vi "MasterAquisitionFile_IOS_postCleanUp.vi"() -> ()   [LabVIEW 2017]
uses:
  <vilib>/userdefined/High Color/IMAQdx.ctl
  <vilib>/vision/driver/IMAQdx.llb/IMAQdx Acquisition Mode.ctl
  <vilib>/vision/driver/IMAQdx.llb/IMAQdx Camera Control Mode.ctl
  <vilib>/vision/driver/IMAQdx.llb/IMAQdx Buffer Number Mode.ctl
  <vilib>/DAQmx/write.llb/DAQmx Write (Digital Bool 1Line 1Point).vi
  <vilib>/DAQmx/read.llb/DAQmx Read (Analog 1D Wfm NChan NSamp).vi
  <vilib>/DAQmx/write.llb/DAQmx Write (Digital 1D Bool NChan 1Samp 1Line).vi
  <vilib>/DAQmx/create/channels.llb/DAQmx Create Channel (DO-Digital Output).vi
  <vilib>/DAQmx/create/channels.llb/DAQmx Create Channel (CO-Pulse Generation-Frequency).vi
  <vilib>/DAQmx/configure/timing.llb/DAQmx Timing (Implicit).vi
  <vilib>/DAQmx/create/channels.llb/DAQmx Create Channel (AI-Voltage-Basic).vi
  <vilib>/DAQmx/configure/timing.llb/DAQmx Timing (Sample Clock).vi
  <vilib>/DAQmx/configure/trigger.llb/DAQmx Start Trigger (Digital Edge).vi
  <vilib>/DAQmx/miscellaneous.llb/DAQmx Fill In Error Info.vi
  <vilib>/vision/driver/NI_Vision_Acquisition_Software.lvlib
  <resource>/objmgr/imaqdx.rc
panel:
  in  "Exposure Time (microsec)":string="10000"
  out "Dropped Frame Table":string[][](table)=[["1236", "1"], ["15481", "1"], ["43559", "1"]]
  out "Solenoids":bool[](array[boolean])
  out "Whisker Camera":bool
  out "Analog Data":bool
  out "Analog acquisition length":i32=61960
  in  "Channel Labels":string[](array[string])=["Neural_LH", "Force_Sensor", "Solenoid_LeftPad", "Solenoid_RightPad", "Solenoid_Auditory", "Respiration", "EMG", "Neural_RH"]
  in  "physical channels":tag="Dev1/ai0:7"
  in  "Whisker Cam ID":T1="cam0"
  in  "WebCam ID":T1="cam3"
  in  "Analog Acquisition":cluster{"Analog Sampling Rate":u16}={"Analog Sampling Rate"=20000} {"Analog Sampling Rate" format="%0.0f"}
  in  "Camera Acquisition Setup":T2={"CBVCam Rate"=30, "WhiskerCam Rate"=150, "WebCam Rate"=15}
  out "Notes Size":i32=7
  out "Notes Reversed":string[](array[string])=["Experimenter", "Animal ID", "Imaged Hemisphere", "Solenoid Pressure", "Isoflurane time", "Session ID", "Amplifier Gain"]
  out "Notes Array":string[](array[string])=["Amplifier Gain", "Session ID", "Isoflurane time", "Solenoid Pressure", "Imaged Hemisphere", "Animal ID", "Experimenter"]
  in  "Session Notes:":T3={"Experimenter"="Kevin", "Animal ID"="T70", "Imaged Hemisphere"="Both", "Solenoid Pressure"="10", "Isoflurane time"="1350", "Session ID"="ImagingSessionOne", "Amplifier Gain"="10000"}
  in  "WhiskCam Trig Source":tag="Dev1/ctr1"
  in  "CBV Cam Trig Source":tag="Dev1/ctr0"
  in  "Left Pad":tag="Dev1/port0/line1"
  in  "Right Pad":tag="Dev1/port0/line0"
  in  "Auditory":tag="Dev1/port0/line3"
  in  "Tail":tag="Dev1/port0/line2"
  in  "Stim Offset (s)":dbl=15.0
  in  "Stim Duration (s)":dbl=0.1 step=0.1
  in  "Inter-Stim Interval (s)":dbl=30.0
  in  "Left Pad":dbl=1.0
  in  "Right Pad":dbl=1.0
  in  "Auditory":dbl=1.0
  in  "Tail":dbl
  in  "Target Path":path=path "C:/Users/klt8/Documents" caption="Final saved file location"
  out "Dropped":u32(slide) caption="Dropped Whisker\nCamera Frames" scale=0.0..50.0
  out "Current file name":string="190407_21_19_47"
  out "Actual WebCam Frame Rate":dbl(knob) scale=0.0..30.0
  out "WebCam":T4(plugin-control)
  out "CBV Camera":bool
  out "Trial Time Elapsed (Min)":cluster{dbl, dbl}(slide)={5.0, 0.051677} scale=0.0..5.0
  in  "Recording Time (min)":dbl(knob)=5.0 min=0.5 max=10.0 step=0.5 scale=0.0..5.0 scale format="%#_2g"
  in  "Temp Path":path=path "C:/Users/klt8/Documents/LabView Test Files" caption="Temporary path for\nstreamed data"
  out "Last CBV\nBuffer":i32=92
  in  "Stop":bool
  out "Actual CBVCam\nFrame Rate":dbl(knob)=30.0 scale=0.0..100.0
  out "Last Whisk\nBuffer":u32=463
  out "Actual WhiskCam\nFrame Rate":dbl(knob)=150.0 scale=0.0..300.0
  # "# Dropped"
  # "Dropped\nIndex"
  # "File Settings:"
  # "Right Pad"
  # "Left Pad"
  # "Tail"
  # "Auditory"
  # "Stimulation Settings:"
  # "Stim. Ratios:"
  # "Output Channels:"
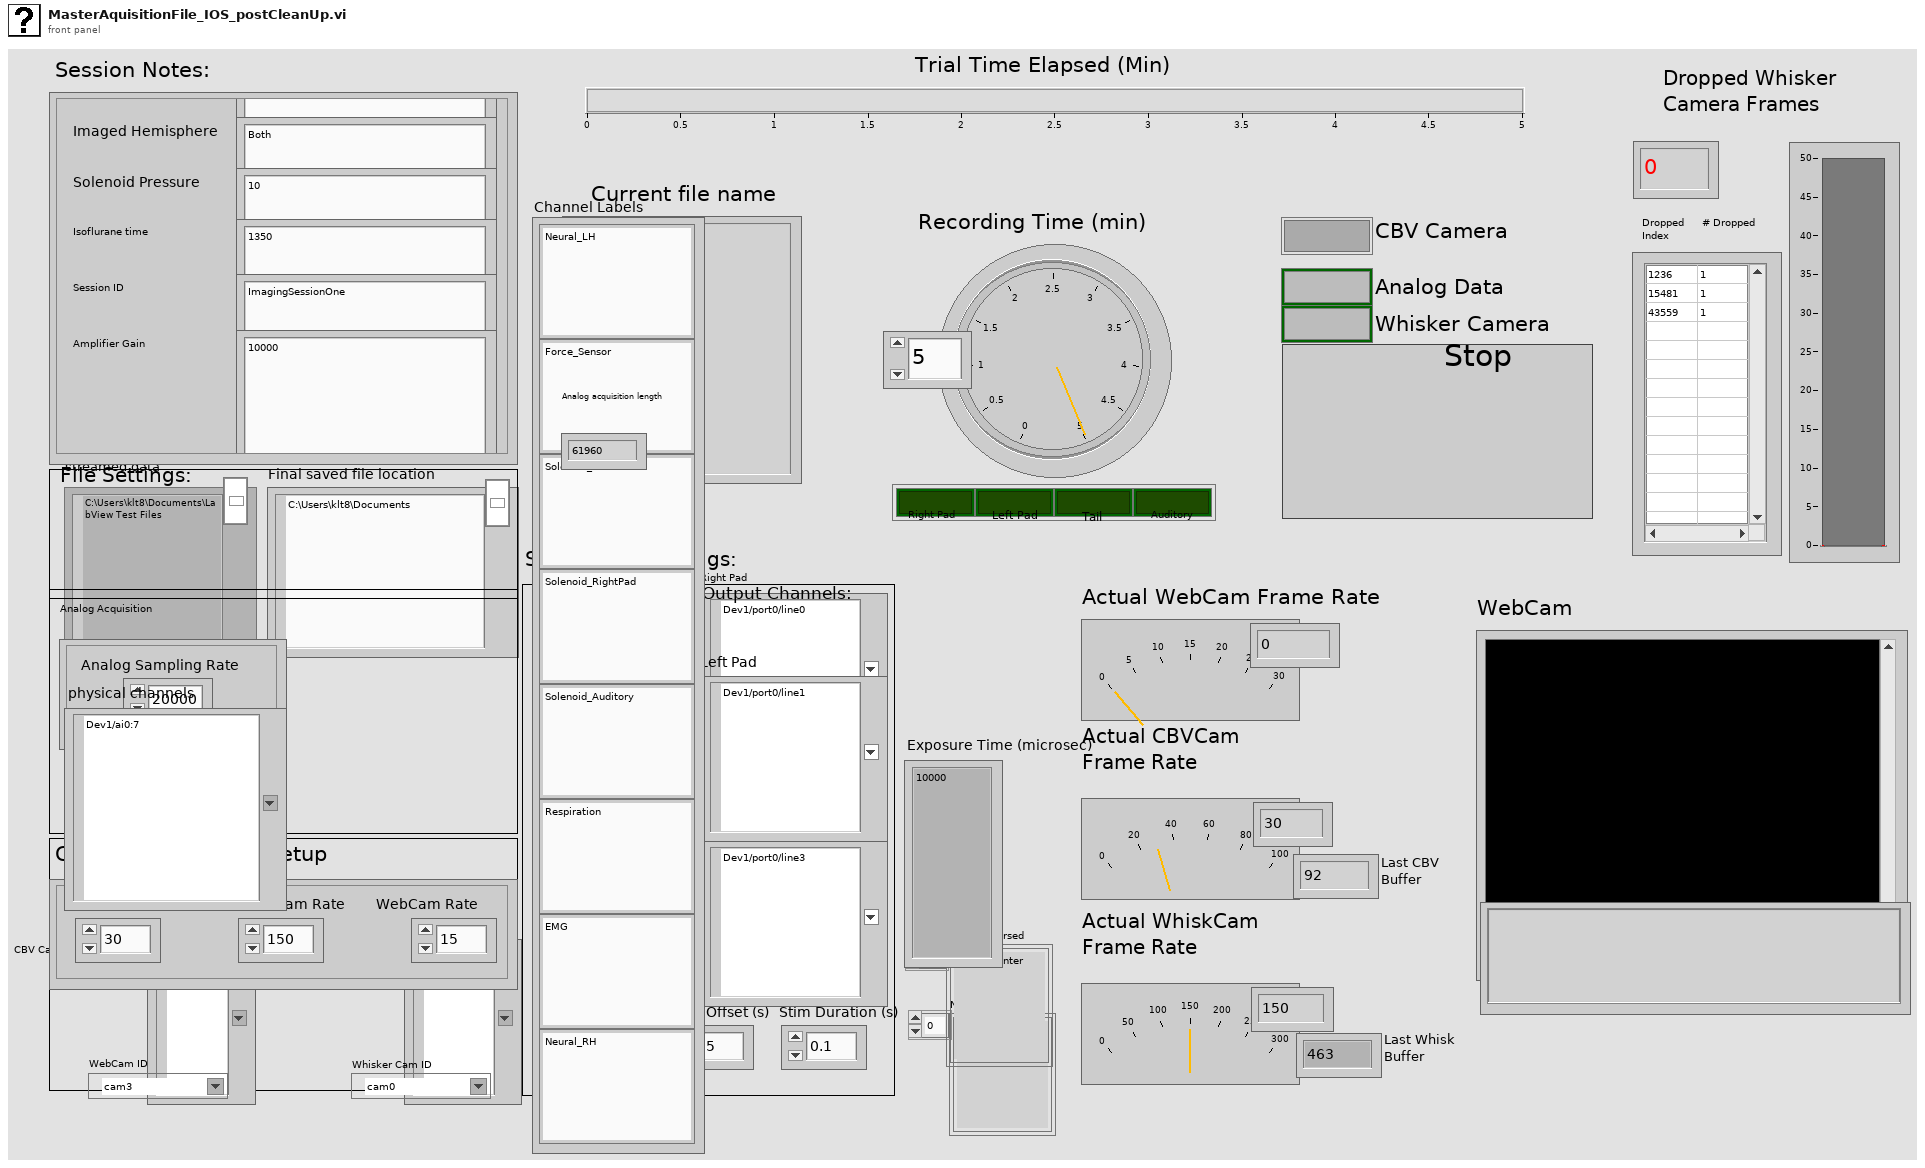
[diagram p1: front panel]
types:
  T1 = typedef "IMAQdx.ctl" = refnum<k21>
  T2 = cluster{"CBVCam Rate":u16, "WhiskerCam Rate":u16, "WebCam Rate":u16}
  T3 = cluster{"Experimenter":string, "Animal ID":string, "Imaged Hemisphere":string, "Solenoid Pressure":string, "Isoflurane time":string, "Session ID":string, "Amplifier Gain":string}
  T4 = typedef "IMAQ Image.ctl" = refnum<image>
  T5 = enum16{"open", "open or create", "create or replace", "create", "open (read-only)"}
  T6 = typedef "Image Type" = u32
  T7 = typedef "NI_Vision_Acquisition_Software.lvlib/IMAQdx Camera Control Mode.ctl" = enum32{"Controller", "Listener"}
  T8 = enum16{"open", "replace", "create", "open or create", "replace or create", "replace or create with confirmation"}
  T9 = typedef "NI_Vision_Acquisition_Software.lvlib/IMAQdx Acquisition Mode.ctl" = enum32{"One Shot", "Continuous"}
  T10 = typedef "IMAQ AVI2 Refnum.ctl" = refnum<k20>
  T11 = enum16{"big-endian, network order", "native, host order", "little-endian"}
  T12 = typedef "NI_Vision_Acquisition_Software.lvlib/IMAQdx Buffer Number Mode.ctl" = enum32{"Next", "Last", "Buffer Number", "Every", "Last New"}
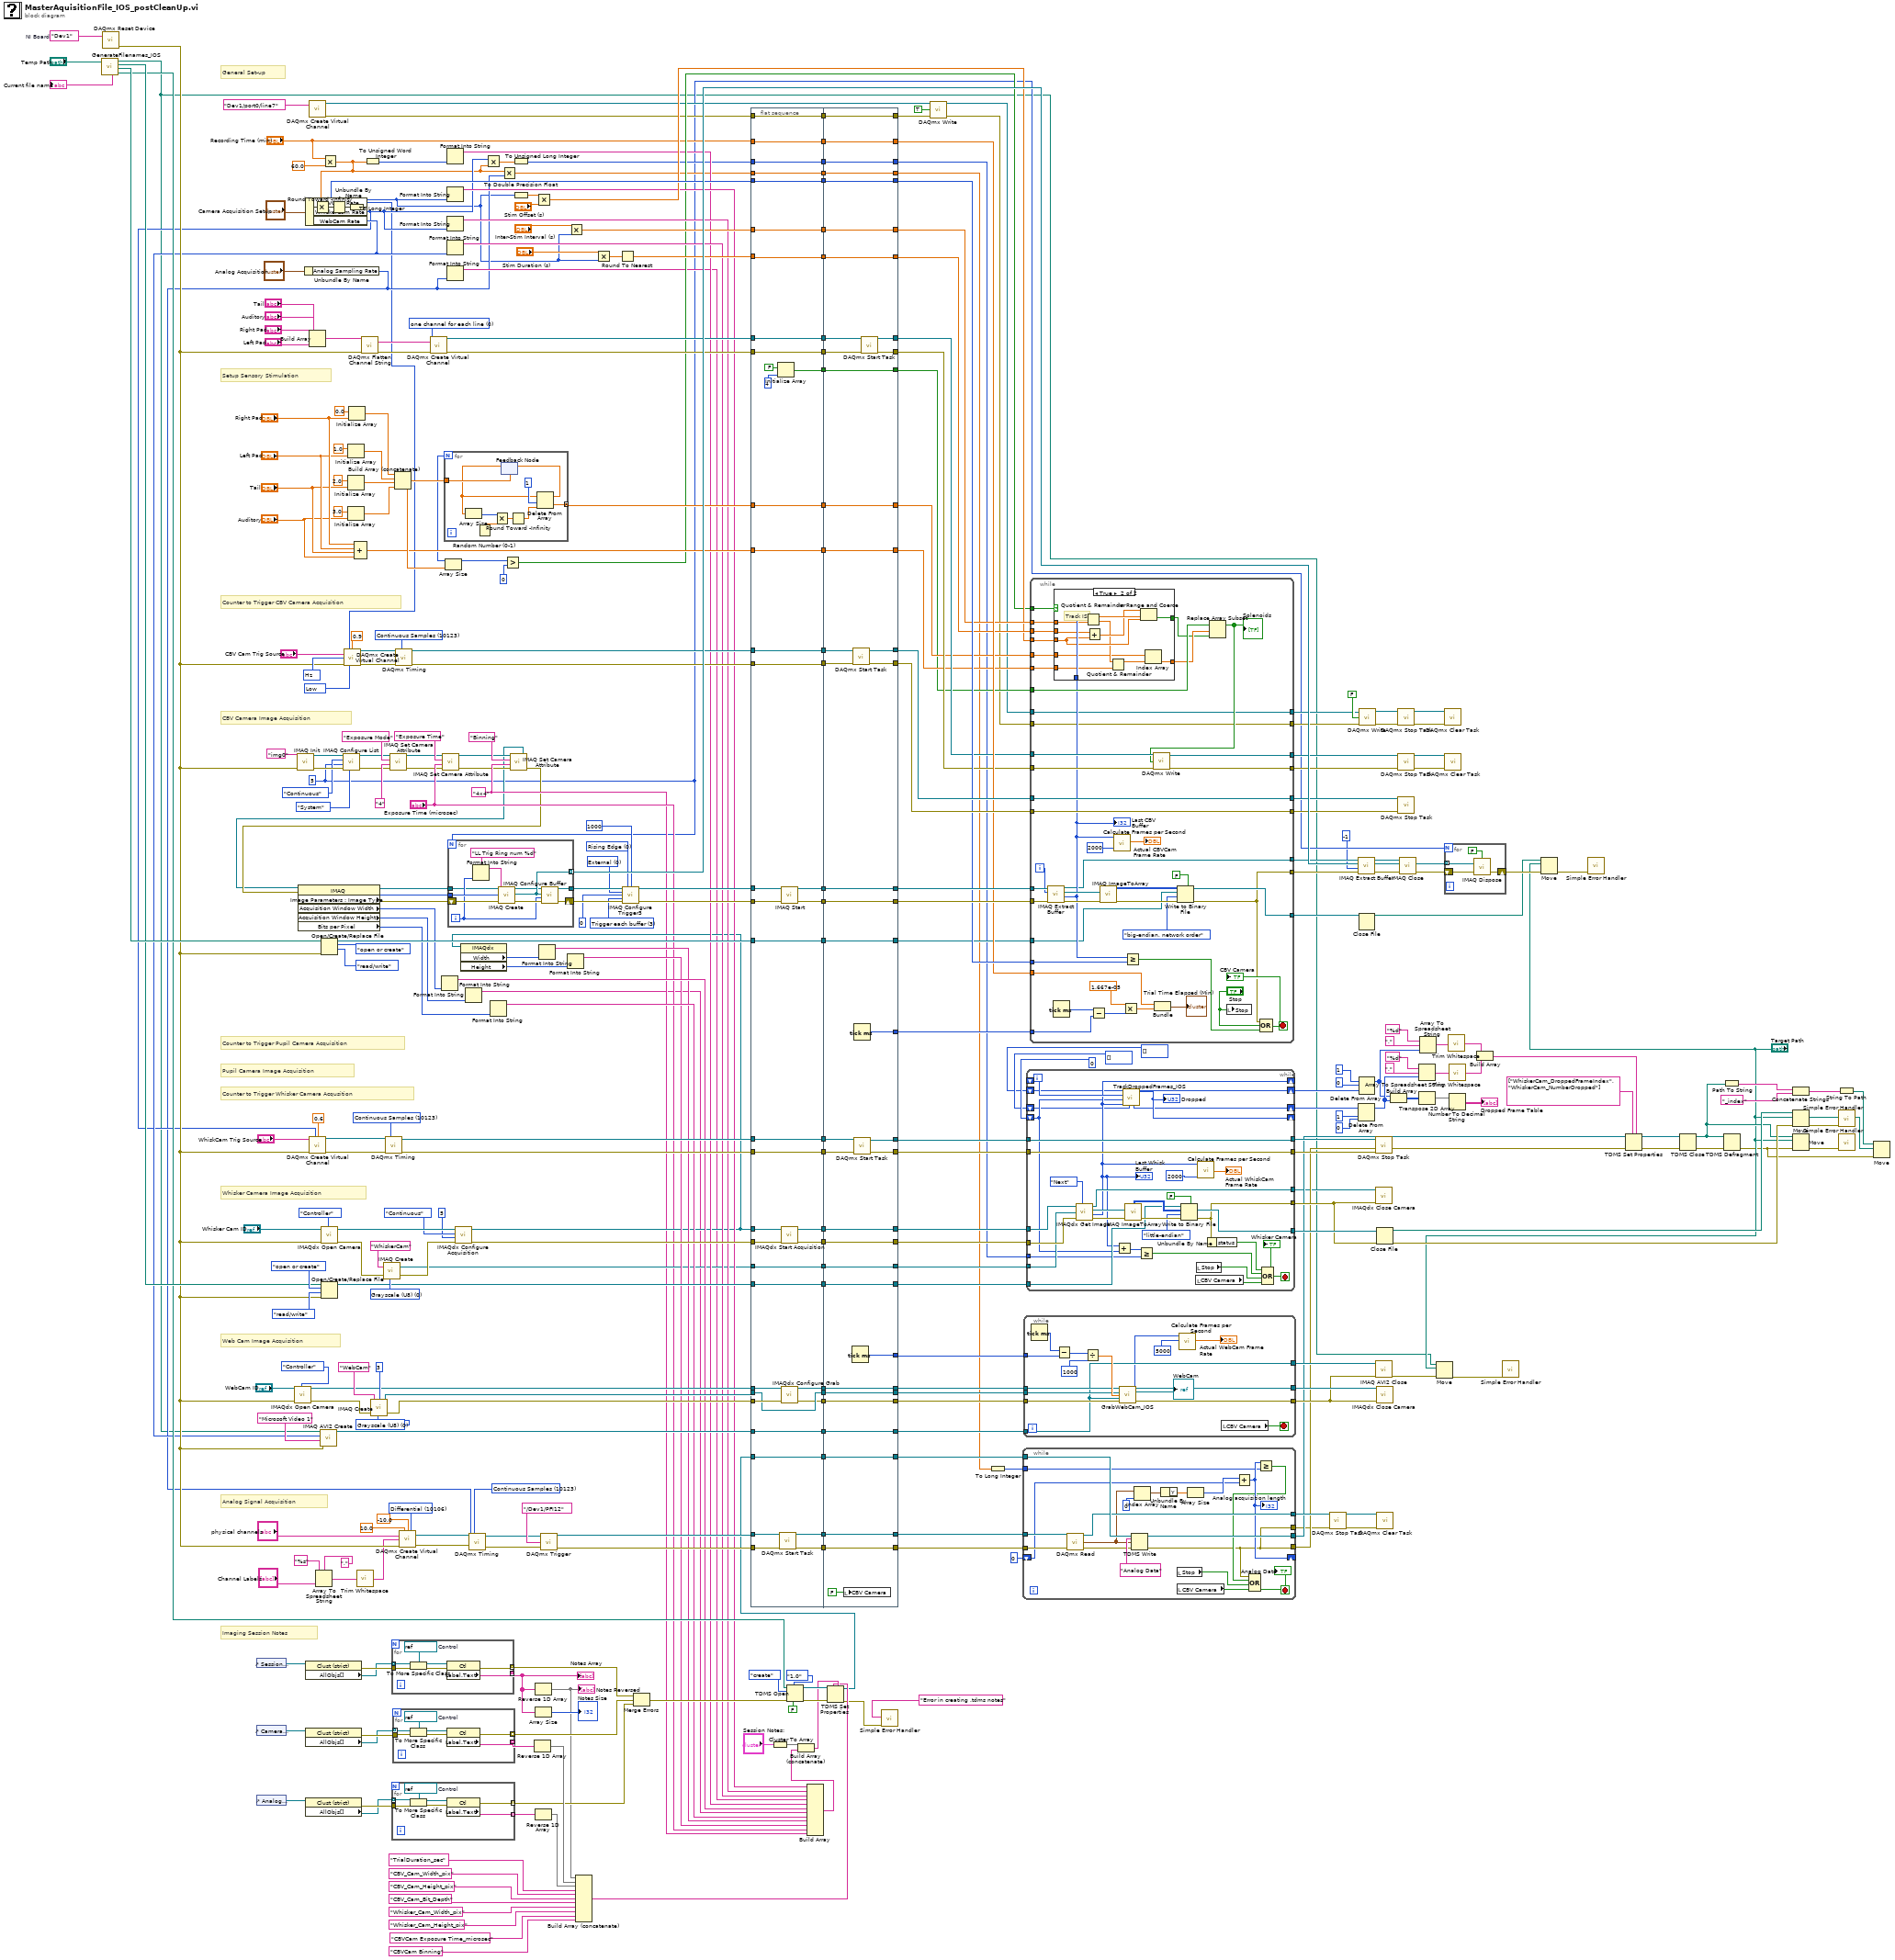
[diagram p0: block diagram]
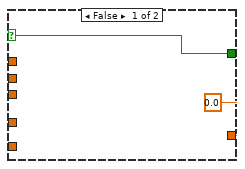
[diagram p2: hidden frame]
diagram:
  w34 = "4x4" ("Attribute Value")
  w195 = 0 items=["one channel for each line", "one channel for all lines"] ("line grouping")
  w252 = 10123 items=["Finite Samples"=10178, "Continuous Samples"=10123, "Hardware Timed Single Point"=12522] ("sample mode")
  w255 = 10106 items=["default"=-1, "RSE"=10083, "NRSE"=10078, "Differential"=10106, "Pseudodifferential"=12529] ("input terminal configuration")
  w309 = T6 0 items=["Grayscale (U8)", "Grayscale (I16)", "Grayscale (SGL)", "Complex (CSG)", "RGB (U32)", "HSL (U32)", "RGB (U64)", "Grayscale (U16)"] ("Image Type")
  w329 = u32 0 items=["Rising Edge", "Falling Edge"] ("Trigger Polarity")
  w332 = u32 0 items=["External"=0, "RTSI"=1, "ISO In"=2, "Scaled Encoder"=5] ("Trigger Type")
  w323 = tag "Dev1"  # NI Board
  w324 = 10123 items=["Finite Samples"=10178, "Continuous Samples"=10123, "Hardware Timed Single Point"=12522] ("sample mode")
  w327 = 10373 items=["Hz"=10373] ("units")
  w328 = 10214 items=["High"=10192, "Low"=10214] ("idle state")
  w5 = u32 5 ("Number of Buffers")
  w330 = u32 3 items=["Disabled", "Trigger start of acquisition", "Trigger start of each buffer list", "Trigger each buffer", "Trigger each line (linescan)", "Trigger end of acquisition"] ("Action")
  w344 = 10123 items=["Finite Samples"=10178, "Continuous Samples"=10123, "Hardware Timed Single Point"=12522] ("sample mode")
  w351 = T6 0 items=["Grayscale (U8)", "Grayscale (I16)", "Grayscale (SGL)", "Complex (CSG)", "RGB (U32)", "HSL (U32)", "RGB (U64)", "Grayscale (U16)"] ("Image Type")
  # "General Set-up"
  # "Pupil Camera Image Acquisition"
  # "Counter to Trigger Pupil Camera Acquisition"
  # "Whisker Camera Image Acquisition"
  # "Imaging Session Notes"
  # "Setup Sensory Stimulation"
  # "CBV Camera Image Acquisition"
  # "Counter to Trigger CBV Camera Acquisition"
  # "Counter to Trigger Whisker Camera Acqusition"
  # "Web Cam Image Acquisition"
  # "Analog Signal Acquisition"
  n1 = call "GenerateFilenames_IOS.vi"("path"="Temp Path") -> ("TDMS Path"=w144:path, "Dalsa Path"=w316:path, "Basler Path"=w312:path, "WebCam Path"=w3:path, "Analog file name"=→"Current file name":string)  [unwired: 5 in, 1 out]
  n2 = call <vilib>:"DAQmx Reset Device.vi"("device in"=w323) -> ("error out"=w149:errorcluster)  [unwired: 14 in]
  n3 = control-ref of="Session Notes:"() -> (w150:refnum<vi>)
  n4 = control-ref of="Camera Acquisition Setup"() -> (w127:refnum<vi>)
  n5 = control-ref of="Analog Acquisition"() -> (w126:refnum<vi>)
  n6 = call <vilib>:"IMAQdx Open Camera.vi"("Camera Control Mode"=IMAQdx_Camera_Control_Mode."Controller", "error in"=w149, "Session In"="WebCam ID") -> ("error out"=w305:errorcluster, "Session Out"=w303:T1)  [unwired: 7 in]
  n7 = call <vilib>:"IMAQ Init.vi"("error in (no error)"=w149, "Interface Name"="img0") -> ("error out"=w342:errorcluster, "IMAQ Session Out"=w343:refnum<k11>)  [unwired: 8 out]
  n8 = Unbundle By Name("Analog Acquisition") -> ("Analog Sampling Rate"=w9:u16)
  n9 = Unbundle By Name("Camera Acquisition Setup") -> ("CBVCam Rate"=w7:u16, "WhiskerCam Rate"=w11:u16, "WebCam Rate"=w120:u16)
  n10 = property class="Clust (strict)"(reference=w150) -> (error out=w153:errorcluster, "AllObjs[]"=w17:refnum<vi>[])  [unwired: 1 in, 1 out]
  n11 = property class="Clust (strict)"(reference=w127) -> (error out=w147:errorcluster, "AllObjs[]"=w18:refnum<vi>[])  [unwired: 1 in, 1 out]
  n12 = property class="Clust (strict)"(reference=w126) -> (error out=w125:errorcluster, "AllObjs[]"=w16:refnum<vi>[])  [unwired: 1 in, 1 out]
  n13 = Build Array("Tail", "Auditory", "Right Pad", "Left Pad") -> (w155:tag[])
  n14 = call-poly <vilib>:"DAQmx Create Virtual Channel.vi"("lines"=tag "Dev1/port0/line7") -> ("task out"=w57:refnum<k21>, "error out"=w60:errorcluster)  [unwired: 13 in]
  n15 = call-poly <vilib>:"DAQmx Create Virtual Channel.vi"("frequency"=w11, "duty cycle"=0.6, "counter"="WhiskCam Trig Source", "error in"=w149) -> ("task out"=w346:refnum<k21>, "error out"=w345:errorcluster)  [unwired: 10 in]
  n16 = Array To Spreadsheet String(delimiter (Tab)=",", array="Channel Labels", 3:"%s" ("format string")) -> (spreadsheet string=w109:string)
  n17 = call "IMAQ AVI2 Create"("error in (no error)"=w149, "Codec"="Microsoft Video 1", "Frames Per Second"=w120, "AVI Path"=w3) -> ("AVI Refnum"=w295:T10)  [unwired: 6 in, 1 out]
  n18 = Open/Create/Replace File(file path (use dialog)=w316, error in=w149, operation (0:open)=T8."open or create", access (0:read/write)=enum16{"read/write", "read-only", "write-only"}."read/write") -> (refnum out=w256:refnum<file>)  [unwired: 2 in, 2 out]
  n19 = Open/Create/Replace File(file path (use dialog)=w312, error in=w149, operation (0:open)=T8."open or create", access (0:read/write)=enum16{"read/write", "read-only", "write-only"}."read/write") -> (refnum out=w275:refnum<file>)  [unwired: 2 in, 2 out]
  n20 = call <vilib>:"IMAQdx Open Camera.vi"("Camera Control Mode"=IMAQdx_Camera_Control_Mode."Controller", "error in"=w149, "Session In"="Whisker Cam ID") -> ("error out"=w354:errorcluster, "Session Out"=w357:T1)  [unwired: 7 in]
  n21 = Multiply(x="Recording Time (min)", y=60.0) -> (x*y=w10:dbl)
  n22 = Multiply(x=w10, y=w7) -> (x*y=w314:dbl)
  n23 = Round Toward -Infinity(1:w314) -> (0:w313:dbl)
  n24 = call <vilib>:"IMAQ Configure List.vi"("Memory Location"=enum16{"System", "Onboard"}."System", "error in (no error)"=w342, "Number of buffers"=w5, "Continuous?"=enum16{"One-Shot", "Continuous"}."Continuous" ("Continuous ?"), "IMAQ Session In"=w343) -> ("error out"=w33:errorcluster, "IMAQ Session Out"=w29:refnum<k11>)  [unwired: 1 in, 4 out]
  n25 = call-poly <vilib>:"DAQmx Create Virtual Channel.vi"("frequency"=w7, "duty cycle"=0.9, "counter"="CBV Cam Trig Source", "units"=w327, "error in"=w149, "idle state"=w328) -> ("task out"=w326:refnum<k21>, "error out"=w325:errorcluster)  [unwired: 8 in]
  n26 = Initialize Array(2.0 ("element"), "Tail") -> (w200:dbl[])
  n27 = Initialize Array(3.0 ("element"), "Auditory") -> (w199:dbl[])
  n28 = Initialize Array(1.0 ("element"), "Left Pad") -> (w201:dbl[])
  n29 = To Long Integer(number=w313) -> (32bit integer=w263:i32)
  n30 = Initialize Array(0.0 ("element"), "Right Pad") -> (w202:dbl[])
  n31 = Compound Arithmetic op=ADD("Right Pad", "Left Pad", "Tail", "Auditory") -> (w179:dbl)
  n32 = call <vilib>:"Trim Whitespace.vi"("string"=w109) -> ("trimmed string"=w108:string)  [unwired: 1 in]
  n33 = call <vilib>:"DAQmx Flatten Channel String.vi"("names in"=w155, "error in"=w149) -> ("names out"=w160:string, "error out"=w154:errorcluster)  [unwired: 12 in]
  n34 = To Unsigned Word Integer(number=w10) -> (unsigned 16bit integer=w103:u16)
  n35 = call "IMAQ Create"("Border Size"=3, "Image Name"="WebCam", "Image Type"=w309, "error in (no error)"=w305) -> ("New Image"=w302:T4, "error out"=w304:errorcluster)  [unwired: 1 in]
  n36 = call "IMAQ Create"("Image Name"="WhiskerCam", "Image Type"=w351, "error in (no error)"=w354) -> ("New Image"=w86:T4, "error out"=w352:errorcluster)  [unwired: 2 in]
  n37 = call-poly <vilib>:"DAQmx Timing.vi"("task/channels in"=w346, "sample mode"=w344, "error in"=w345) -> ("task out"=w235:refnum<k21>, "error out"=w233:errorcluster)  [unwired: 11 in]
  n38 = call <vilib>:"IMAQ Set Camera Attribute.vi"("error in (no error)"=w33, "Attribute Value"="4", "Camera Attribute"="Exposure Mode", "IMAQ Session In"=w29) -> ("error out"=w32:errorcluster, "IMAQ Session Out"=w28:refnum<k11>)  [unwired: 4 in]
  n39 = for {
    tunnel: [w363] -> w152 mode=indexing
    tunnel: w153 -> [w362]
    tunnel: [w360] -> w134 mode=indexing
    tunnel: w17 -> [w359] mode=indexing
    w364 = refnum<vi> refnum  # Control
    n40 = To More Specific Class(target class=w364, reference=w359, error in=w362) -> (specific class reference=w365:refnum<vi>, error out=w361:errorcluster)
    n41 = property class="Ctl"(reference=w365, error in=w361) -> (error out=w360:errorcluster, "Label.Text"=w363:string)  [unwired: 1 out]
  }
  "Notes Array" <- w152
  n42 = for {
    tunnel: [w370] -> w123 mode=indexing
    tunnel: w125 -> [w369]
    tunnel: [w367] -> w124 mode=indexing
    tunnel: w16 -> [w366] mode=indexing
    w371 = refnum<vi> refnum  # Control
    n43 = To More Specific Class(target class=w371, reference=w366, error in=w369) -> (specific class reference=w372:refnum<vi>, error out=w368:errorcluster)
    n44 = property class="Ctl"(reference=w372, error in=w368) -> (error out=w367:errorcluster, "Label.Text"=w370:string)  [unwired: 1 out]
  }
  n45 = for {
    tunnel: [w377] -> w148 mode=indexing
    tunnel: w147 -> [w376]
    tunnel: [w374] -> w133 mode=indexing
    tunnel: w18 -> [w373] mode=indexing
    w378 = refnum<vi> refnum  # Control
    n46 = To More Specific Class(target class=w378, reference=w373, error in=w376) -> (specific class reference=w379:refnum<vi>, error out=w375:errorcluster)
    n47 = property class="Ctl"(reference=w379, error in=w375) -> (error out=w374:errorcluster, "Label.Text"=w377:string)  [unwired: 1 out]
  }
  n48 = Build Array (concatenate)(w202, w201, w200, w199) -> (w198:dbl[])
  n49 = call-poly <vilib>:"DAQmx Timing.vi"("task/channels in"=w326, "sample mode"=w324, "error in"=w325) -> ("task out"=w239:refnum<k21>, "error out"=w237:errorcluster)  [unwired: 11 in]
  n50 = call-poly <vilib>:"DAQmx Create Virtual Channel.vi"("maximum value"=10.0, "minimum value"=-10.0, "input terminal configuration"=w255, "physical channels"="physical channels", "name to assign"=w108, "error in"=w149) -> ("task out"=w254:refnum<k21>, "error out"=w253:errorcluster)  [unwired: 8 in]
  n51 = call-poly <vilib>:"DAQmx Create Virtual Channel.vi"("lines"=w160, "line grouping"=w195, "error in"=w154) -> ("task out"=w193:refnum<k21>, "error out"=w191:errorcluster)  [unwired: 11 in]
  n52 = call <vilib>:"IMAQ Set Camera Attribute.vi"("error in (no error)"=w32, "Attribute Value"="Exposure Time (microsec)", "Camera Attribute"="Exposure Time", "IMAQ Session In"=w28) -> ("error out"=w31:errorcluster, "IMAQ Session Out"=w27:refnum<k11>)  [unwired: 4 in]
  n53 = Array Size(array=w198) -> (size(s)=w114:i32)
  n54 = for {
    N: w114 -> [_]
    tunnel: w198 -> [w383]
    tunnel: [w380] -> w176 mode=concatenating
    n55 = Random Number (0-1)() -> (number: 0 to 1=w387:dbl)
    n56 = feedback #1(w383) -> (w382:dbl[])
    n57 = Array Size(array=w382) -> (size(s)=w388:i32)
    n58 = Multiply(x=w388, y=w387) -> (x*y=w386:dbl)
    n59 = Round Toward -Infinity(1:w386) -> (0:w385:dbl)
    n60 = Delete From Array(array=w382, length=1, index=w385) -> (deleted portion=w380:dbl[], array with subset deleted=w381:dbl[])
    n61 = feedback-in #1(w381) -> ()
  }
  n62 = Format Into String(w103) -> (resulting string=w105:string)  [unwired: 3 in, 1 out]
  n63 = Format Into String(w7) -> (resulting string=w119:string)  [unwired: 3 in, 1 out]
  n64 = Format Into String(w11) -> (resulting string=w118:string)  [unwired: 3 in, 1 out]
  n65 = Format Into String(w120) -> (resulting string=w117:string)  [unwired: 3 in, 1 out]
  n66 = Format Into String(w9) -> (resulting string=w13:string)  [unwired: 3 in, 1 out]
  n67 = call <vilib>:"IMAQdx Configure Acquisition.vi"("error in"=w352, "Number of Buffers"=u32 5, "Continuous?"=IMAQdx_Acquisition_Mode."Continuous", "Session In"=w357) -> ("error out"=w284:errorcluster, "Session Out"=w87:T1)  [unwired: 6 in]
  n68 = property class="IMAQdx"(reference=w87) -> ("Width"=w102:u32, "Height"=w101:u32)  [unwired: 1 in, 2 out]
  n69 = call-poly <vilib>:"DAQmx Timing.vi"("task/channels in"=w254, "sample mode"=w252, "rate"=w9, "error in"=w253) -> ("task out"=w14:refnum<k21>, "error out"=w251:errorcluster)  [unwired: 10 in]
  n70 = Multiply(x=w11, y=w10) -> (x*y=w8:dbl)
  n71 = Multiply(x=w10, y=w9) -> (x*y=w68:dbl)
  n72 = Greater?(x=w114, y=0) -> (0:w112:bool)
  n73 = call <vilib>:"IMAQ Set Camera Attribute.vi"("error in (no error)"=w31, "Attribute Value"=w34, "Camera Attribute"="Binning", "IMAQ Session In"=w27) -> ("error out"=w30:errorcluster, "IMAQ Session Out"=w26:refnum<k11>)  [unwired: 4 in]
  n74 = property class="IMAQ"(reference=w26, error in=w30) -> (reference out=w43:refnum<k11>, error out=w42:errorcluster, "Image Parameters : Image Type"=w338:u32, "Acquisition Window Width"=w100:u32, "Acquisition Window Height"=w99:u32, "Bits per Pixel"=w98:u32)
  n75 = Format Into String(w100) -> (resulting string=w97:string)  [unwired: 3 in, 1 out]
  n76 = for {
    N: w5 -> [_]
    tunnel: [w398] -> w334
    tunnel: w338 -> [w396]
    shift-right: [w397] -> w333
    shift-left: w42 -> [w395]
    tunnel: [w390] -> w335 mode=indexing
    tunnel: w43 -> [w389]
    i -> [w391]
    n77 = Format Into String(format string="LL Trig Ring num %d", w391) -> (resulting string=w393:string)  [unwired: 2 in, 1 out]
    n78 = call "IMAQ Create"("Image Name"=w393, "Image Type"=w396, "error in (no error)"=w395) -> ("New Image"=w390:T4, "error out"=w394:errorcluster)  [unwired: 1 in, 1 out]
    n79 = call <vilib>:"IMAQ Configure Buffer.vi"("error in (no error)"=w394, "Buffer Number"=w391, "Image In"=w390, "IMAQ Session In"=w389) -> ("error out"=w397:errorcluster, "IMAQ Session Out"=w398:refnum<k11>)  [unwired: 2 in, 4 out]
  }
  n80 = Format Into String(w99) -> (resulting string=w6:string)  [unwired: 3 in, 1 out]
  n81 = Format Into String(w98) -> (resulting string=w96:string)  [unwired: 3 in, 1 out]
  n82 = To Unsigned Long Integer(number=w8) -> (unsigned 32bit integer=w65:u32)
  n83 = To Double Precision Float(number=w7) -> (double precision float=w161:dbl)
  n84 = Reverse 1D Array(array=w148) -> (reversed array=w138:string[])
  n85 = Reverse 1D Array(array=w152) -> (reversed array=w15:string[])
  "Notes Reversed" <- w15
  n86 = Array Size(array=w152) -> (size(s)=→"Notes Size":i32)
  n87 = Reverse 1D Array(array=w123) -> (reversed array=w122:string[])
  n88 = Multiply(x="Stim Offset (s)", y=w161) -> (x*y=w162:dbl)
  n89 = Format Into String(w102) -> (resulting string=w95:string)  [unwired: 3 in, 1 out]
  n90 = call-poly <vilib>:"DAQmx Trigger.vi"("task/channels in"=w14, "source"=tag "/Dev1/PFI12", "error in"=w251) -> ("task out"=w249:refnum<k21>, "error out"=w248:errorcluster)  [unwired: 11 in]
  n91 = Format Into String(w101) -> (resulting string=w94:string)  [unwired: 3 in, 1 out]
  n92 = Multiply(x="Inter-Stim Interval (s)", y=w7) -> (x*y=w183:dbl)
  n93 = Build Array (concatenate)(w15, w138, w122, "TrialDuration_sec", "CBV_Cam_Width_pix", "CBV_Cam_Height_pix", "CBV_Cam_Bit_Depth", "Whisker_Cam_Width_pix", "Whisker_Cam_Height_pix", "CBVCam Exposure Time_microsec" ("element"), "CBVCam Binning" ("element")) -> (w136:string[])
  n94 = Multiply(x="Stim Duration (s)", y=w7) -> (x*y=w170:dbl)
  n95 = Round To Nearest(number=w170) -> (nearest integer value=w169:dbl)
  n96 = call <vilib>:"IMAQ Configure Trigger3.vi"("IMAQ Session In"=w334, "Polarity"=w329, "Frame timeout (ms)"=u32 1000 ("Frame Timeout (ms)"), "Type"=w332, "Line Number"=u32 0 ("Trigger Line Number"), "Action"=w330, "error in (no error)"=w333) -> ("IMAQ Session Out"=w274:refnum<k11>, "error out"=w273:errorcluster)  [unwired: 2 in, 5 out]
  n97 = Merge Errors(w134, w133, w124) -> (w132:errorcluster)
  n98 = flat-sequence {
    tunnel: w304 -> [w438]
    tunnel: w303 -> [w437]
    tunnel: w302 -> [w436]
    tunnel: [w436] -> w301
    tunnel: [w435] -> w299
    tunnel: [w434] -> w297
    tunnel: w295 -> [w433]
    tunnel: [w433] -> w294
    tunnel: w87 -> [w432]
    tunnel: w284 -> [w431]
    tunnel: [w430] -> w282
    tunnel: [w429] -> w280
    tunnel: [w428] -> w278
    tunnel: w86 -> [w428]
    tunnel: [w427] -> w276
    tunnel: w275 -> [w427]
    tunnel: w274 -> [w426]
    tunnel: w273 -> [w425]
    tunnel: [w424] -> w271
    tunnel: [w423] -> w269
    tunnel: w263 -> [w422]
    tunnel: [w422] -> w262
    tunnel: "Recording Time (min)" -> [w421]
    tunnel: [w421] -> w259
    tunnel: [w420] -> w257
    tunnel: w256 -> [w420]
    tunnel: w249 -> [w419]
    tunnel: w248 -> [w418]
    tunnel: [w417] -> w247
    tunnel: [w416] -> w246
    tunnel: [w415] -> w241
    tunnel: w135 -> [w415]
    tunnel: w239 -> [w414]
    tunnel: [w414] -> w238
    tunnel: w237 -> [w413]
    tunnel: [w413] -> w236
    tunnel: w235 -> [w412]
    tunnel: [w412] -> w234
    tunnel: w233 -> [w411]
    tunnel: [w411] -> w232
    tunnel: w193 -> [w410]
    tunnel: [w410] -> w194
    tunnel: w191 -> [w409]
    tunnel: [w409] -> w192
    tunnel: w183 -> [w408]
    tunnel: [w408] -> w182
    tunnel: [w407] -> w180
    tunnel: w169 -> [w407]
    tunnel: w179 -> [w406]
    tunnel: [w406] -> w178
    tunnel: w176 -> [w405]
    tunnel: [w405] -> w175
    tunnel: [w403] -> w173
    tunnel: w68 -> [w401]
    tunnel: [w401] -> w67
    tunnel: w65 -> [w400]
    tunnel: [w400] -> w64
    tunnel: w60 -> [w399]
    tunnel: [w399] -> w59
    tunnel: [w477] -> w306
    tunnel: w301 -> [w476]
    tunnel: [w476] -> w300
    tunnel: w299 -> [w475]
    tunnel: [w475] -> w298
    tunnel: w297 -> [w474]
    tunnel: [w474] -> w296
    tunnel: w294 -> [w473]
    tunnel: [w473] -> w293
    tunnel: [w455] -> w289
    tunnel: [w454] -> w287
    tunnel: [w472] -> w283
    tunnel: w282 -> [w472]
    tunnel: [w471] -> w281
    tunnel: w280 -> [w471]
    tunnel: [w470] -> w279
    tunnel: w278 -> [w470]
    tunnel: [w469] -> w277
    tunnel: w276 -> [w469]
    tunnel: [w468] -> w272
    tunnel: w271 -> [w468]
    tunnel: [w467] -> w270
    tunnel: w269 -> [w467]
    tunnel: [w459] -> w267
    tunnel: [w458] -> w265
    tunnel: [w466] -> w264
    tunnel: w262 -> [w465]
    tunnel: [w465] -> w261
    tunnel: [w464] -> w260
    tunnel: w259 -> [w464]
    tunnel: [w463] -> w258
    tunnel: w257 -> [w463]
    tunnel: [w462] -> w244
    tunnel: w247 -> [w462]
    tunnel: [w461] -> w245
    tunnel: w246 -> [w461]
    tunnel: [w460] -> w242
    tunnel: w241 -> [w460]
    tunnel: w238 -> [w457]
    tunnel: w236 -> [w456]
    tunnel: w234 -> [w453]
    tunnel: w232 -> [w452]
    tunnel: w194 -> [w451]
    tunnel: w192 -> [w450]
    tunnel: [w449] -> w190
    tunnel: [w448] -> w189
    tunnel: [w447] -> w184
    tunnel: w182 -> [w447]
    tunnel: [w446] -> w181
    tunnel: w180 -> [w446]
    tunnel: w178 -> [w445]
    tunnel: [w445] -> w177
    tunnel: w175 -> [w444]
    tunnel: [w444] -> w174
    tunnel: w173 -> [w443]
    tunnel: [w443] -> w172
    tunnel: w67 -> [w442]
    tunnel: [w442] -> w4
    tunnel: w64 -> [w441]
    tunnel: [w441] -> w63
    tunnel: w59 -> [w440]
    tunnel: [w440] -> w58
    frame #0 {
      n99 = Initialize Array(FALSE, 4 ("dimension size")) -> (w403:bool[])
      n100 = call <vilib>:"DAQmx Start Task.vi"("task/channels in"=w419, "error in"=w418) -> ("task out"=w417:refnum<k21>, "error out"=w416:errorcluster)  [unwired: 12 in]
      n101 = call <vilib>:"IMAQdx Configure Grab.vi"("error in"=w438, "Session In"=w437) -> ("error out"=w434:errorcluster, "Session Out"=w435:T1)  [unwired: 8 in]
      n102 = call <vilib>:"IMAQ Start.vi"("error in (no error)"=w425, "IMAQ Session In"=w426) -> ("error out"=w423:errorcluster, "IMAQ Session Out"=w424:refnum<k11>)  [unwired: 8 out]
      n103 = call <vilib>:"IMAQdx Start Acquisition.vi"("error in"=w431, "Session In"=w432) -> ("error out"=w429:errorcluster, "Session Out"=w430:T1)  [unwired: 8 in]
    }
    frame #1 {
      n104 = local write "CBV Camera"(FALSE ("Finished Acquiring")) -> ()
      n105 = Tick Count (ms)() -> (millisecond timer value=w477:u32)
      n106 = call <vilib>:"DAQmx Start Task.vi"("task/channels in"=w457, "error in"=w456) -> ("task out"=w459:refnum<k21>, "error out"=w458:errorcluster)  [unwired: 12 in]
      n107 = call <vilib>:"DAQmx Start Task.vi"("task/channels in"=w453, "error in"=w452) -> ("task out"=w455:refnum<k21>, "error out"=w454:errorcluster)  [unwired: 12 in]
      n108 = Tick Count (ms)() -> (millisecond timer value=w466:u32)
      n109 = call <vilib>:"DAQmx Start Task.vi"("task/channels in"=w451, "error in"=w450) -> ("task out"=w449:refnum<k21>, "error out"=w448:errorcluster)  [unwired: 12 in]
    }
  }
  n110 = Cluster To Array(cluster="Session Notes:") -> (array=w145:string[])
  n111 = TDMS Open(6:FALSE ("disable buffering? (T)"), 7:enum16{"1.0", "2.0"}."1.0" ("file format version (2.0)"), 8:w132, 10:T5."create" ("operation (0:open)"), 11:w144) -> (0:w139:errorcluster, 3:w140:refnum<k34>)  [unwired: 2 in]
  n112 = Build Array(w119, w118, w117, w13, w105, w97, w6, w96, w95, w94, "Exposure Time (microsec)", w34) -> (w116:string[])
  n113 = Build Array (concatenate)(w145, w116) -> (w137:string[])
  n114 = TDMS Set Properties(5:w137, 7:w136, 8:w139, 11:w140) -> (0:w131:errorcluster, 3:w135:refnum<k34>)  [unwired: 2 in, 2 out]
  n115 = call <vilib>:"Simple Error Handler.vi"("error source (\" \")"="Error in creating .tdms notes" ("error source (\" \")"), "error in (no error)"=w131) -> ()  [unwired: 3 in, 5 out]
  n116 = call-poly <vilib>:"DAQmx Write.vi"("task/channels in"=w57, "data"=TRUE, "error in"=w58) -> ("task out"=w55:refnum<k21>, "error out"=w53:errorcluster)  [unwired: 10 in, 1 out]
  n117 = To Long Integer(number=w4) -> (32bit integer=w66:i32)
  n118 = while {
    tunnel: w245 -> [w497]
    tunnel: w244 -> [w496]
    tunnel: w242 -> [w495]
    tunnel: [w494] -> w85
    tunnel: [w478] -> w84
    tunnel: [w493] -> w240
    shift-right: [w485] -> _
    shift-left: 0 -> [w486]
    tunnel: w66 -> [w484]
    tunnel: [w478] -> w1
    stop <- w480 stop-if-true
    n119 = call-poly <vilib>:"DAQmx Read.vi"("task/channels in"=w496, "error in"=w497) -> ("task out"=w493:refnum<k21>, "data"=w491:waveform(dbl)[], "error out"=w483:errorcluster)  [unwired: 11 in]
    n120 = TDMS Write(0:w495, 5:"Analog Data" ("group name in (Untitled)"), 9:w491, 11:w483) -> (4:w494:refnum<k34>, 15:w478:errorcluster)  [unwired: 2 in, 2 out]
    n121 = Index Array(array=w491, index=0) -> (element=w489:waveform(dbl))
    n122 = Unbundle By Name(w489) -> ("Y"=w488:dbl[])
    n123 = local read "Stop"() -> (w481:bool)
    n124 = local read "CBV Camera"() -> (w479:bool)
    n125 = Array Size(array=w488) -> (size(s)=w487:i32)
    n126 = Add(x=w487, y=w486) -> (x+y=w485:i32)
    "Analog acquisition length" <- w485
    n127 = Greater Or Equal?(x=w485, y=w484) -> (x >= y?=w482:bool)
    n128 = Compound Arithmetic op=OR(w478, w482, w481, w479) -> (w480:bool)
    "Analog Data" <- w480
  }
  n129 = while {
    tunnel: w306 -> [w507]
    tunnel: w300 -> [w505]
    tunnel: w298 -> [w504]
    tunnel: w296 -> [w503]
    tunnel: w293 -> [w499]
    tunnel: [w501] -> w292
    tunnel: [w500] -> w290
    tunnel: [w499] -> w291
    stop <- w510 stop-if-true
    n130 = Tick Count (ms)() -> (millisecond timer value=w511:u32)
    n131 = Subtract(x=w511, y=w507) -> (x-y=w512:u32)
    n132 = Divide(x=w512, y=u32 1000) -> (x/y=w506:dbl)
    n133 = call "GrabWebCam_IOS.vi"("Session In"=w504, "Image In"=w505, "Trial Time"=w506, "AVI Refnum"=w499, "error in"=w503) -> ("Session Out"=w501:T1, "WebCam Img Out"=→"WebCam":T4, "Buffer Number Out"=w498:u32, "error out"=w500:errorcluster)  [unwired: 7 in]
    n134 = call <vilib>:"Calculate Frames per Second.vi"("Update Interval (ms)"=u32 5000, "Buffer Number"=w498) -> ("Processed Frames/s"=→"Actual WebCam Frame Rate":dbl)  [unwired: 7 in, 2 out]
    n135 = local read "CBV Camera"() -> (w510:bool)
  }
  n136 = while {
    tunnel: w289 -> [w536]
    tunnel: [w537] -> w288
    tunnel: w287 -> [w537]
    tunnel: [w536] -> w286
    tunnel: [w525] -> w81
    tunnel: [w526] -> w163
    tunnel: [w535] -> w285
    tunnel: w283 -> [w534]
    tunnel: w281 -> [w533]
    tunnel: w279 -> [w532]
    tunnel: w277 -> [w531]
    shift-right: [w524] -> _
    shift-left: _ -> [w530]
    shift-right: [w529] -> _
    shift-left: u32 0 ("New Lost") -> [w523]
    shift-right: [w528] -> w70
    shift-left: u32[] [] ("NewBuffNum") -> [w514]
    shift-right: [w527] -> w226
    shift-left: u32[] [] ("NewNumLost") -> [w515]
    tunnel: w63 -> [w521]
    stop <- w517 stop-if-true
    n137 = call <vilib>:"IMAQdx Get Image.vi"("Buffer Number Mode (Next)"=IMAQdx_Buffer_Number_Mode."Next", "error in"=w533, "Image In"=w532, "Session In"=w534) -> ("error out"=w545:errorcluster, "Buffer Number Out"=w524:u32, "Image Out"=w544:T4, "Session Out"=w525:T1)  [unwired: 4 in]
    "Last Whisk\nBuffer" <- w524
    n138 = Add(x=w524, y=w523) -> (x+y=w522:u32)
    n139 = call "TrackDroppedFrames_IOS.vi"("NumLost"=w515, "BuffNum"=w514, "Curr Buffer"=w524, "Prev Lost"=w523, "Prev Buffer"=w530) -> ("New Lost"=w529:u32, "NewNumLost"=w527:u32[], "NewBuffNum"=w528:u32[])  [unwired: 4 in]
    "Dropped" <- w529
    n140 = call "IMAQ ImageToArray"("error in (no error)"=w545, "Image"=w544) -> ("error out"=w543:errorcluster, "Image Pixels (U8)"=w542:u8[][])  [unwired: 2 in, 3 out]
    n141 = Greater Or Equal?(x=w522, y=w521) -> (x >= y?=w519:bool)
    n142 = Write to Binary File(file (use dialog)=w531, data=w542, error in=w543, 5:FALSE ("prepend array or string size? (T)"), 9:T11."little-endian" ("byte order (0:big-endian, network order)")) -> (refnum out=w535:refnum<file>, error out=w526:errorcluster)  [unwired: 1 in, 1 out]
    n143 = local read "CBV Camera"() -> (w516:bool)
    n144 = local read "Stop"() -> (w518:bool)
    n145 = call <vilib>:"Calculate Frames per Second.vi"("Update Interval (ms)"=u32 2000, "Buffer Number"=w524) -> ("Processed Frames/s"=→"Actual WhiskCam\nFrame Rate":dbl)  [unwired: 7 in, 2 out]
    n146 = Unbundle By Name(w526) -> ("status"=w520:bool)
    n147 = Compound Arithmetic op=OR(w520, w519, w518, w516) -> (w517:bool)
    "Whisker Camera" <- w517
  }
  n148 = while {
    tunnel: w272 -> [w590]
    tunnel: w270 -> [w591]
    tunnel: [w550] -> w318
    tunnel: [w548] -> w319
    tunnel: [w582] -> w317
    tunnel: [w576] -> w268
    tunnel: w267 -> [w576]
    tunnel: [w575] -> w266
    tunnel: w265 -> [w575]
    tunnel: w264 -> [w574]
    tunnel: w261 -> [w573]
    tunnel: w260 -> [w572]
    tunnel: w258 -> [w547]
    tunnel: w190 -> [w569]
    tunnel: w189 -> [w568]
    tunnel: [w567] -> w188
    tunnel: [w566] -> w187
    tunnel: w184 -> [w561]
    tunnel: w181 -> [w560]
    tunnel: w177 -> [w558]
    tunnel: w174 -> [w556]
    tunnel: w172 -> [w565]
    tunnel: w162 -> [w559]
    tunnel: w112 -> [w563]
    tunnel: w55 -> [w552]
    tunnel: [w552] -> w54
    tunnel: [w551] -> w52
    tunnel: w53 -> [w551]
    i -> [w589]
    stop <- w554 stop-if-true
    # "Track ISI"
    n149 = call <vilib>:"IMAQ Extract Buffer.vi"("error in (no error)"=w591, "Buffer to extract"=w589, "IMAQ Session In"=w590) -> ("error out"=w581:errorcluster, "Buffer Number"=w562:i32, "Image Out"=w587:T4, "IMAQ Session Out"=w548:refnum<k11>)  [unwired: 5 out]
    "Last CBV\nBuffer" <- w562
    n150 = Tick Count (ms)() -> (millisecond timer value=w580:u32)
    n151 = case shown="True" w563 {
      selector: w563 -> [w593 _]
      tunnel: w562 -> [_ w603]
      tunnel: w561 -> [_ w602]
      tunnel: w560 -> [_ w601]
      tunnel: w559 -> [_ w600]
      tunnel: w558 -> [_ w597]
      tunnel: [0.0 ("element") w594] -> w557
      tunnel: w556 -> [_ w596]
      tunnel: [w593 w595] -> w555
      frame False {
      }
      frame True {
        n152 = Quotient & Remainder(x=w603, y=w602) -> (x-y*floor(x/y)=w605:dbl, floor(x/y)=w598:dbl)
        n153 = Add(x=w601, y=w600) -> (x+y=w604:dbl)
        n154 = Quotient & Remainder(x=w598, y=w597) -> (x-y*floor(x/y)=w599:dbl)  [unwired: 1 out]
        n155 = In Range and Coerce(upper limit=w604, x=w605, lower limit=w600) -> (In Range?=w595:bool)  [unwired: 1 out]
        n156 = Index Array(array=w596, index=w599) -> (element=w594:dbl)
      }
    }
    n157 = Subtract(x=w580, y=w574) -> (x-y=w579:u32)
    n158 = call "IMAQ ImageToArray"("error in (no error)"=w581, "Image"=w587) -> ("error out"=w586:errorcluster, "Image Pixels (I16)"=w585:i16[][])  [unwired: 2 in, 3 out]
    n159 = call <vilib>:"Calculate Frames per Second.vi"("Update Interval (ms)"=u32 2000, "Buffer Number"=w562) -> ("Processed Frames/s"=→"Actual CBVCam\nFrame Rate":dbl)  [unwired: 7 in, 2 out]
    n160 = Multiply(x=w579, y=1.667e-05) -> (x*y=w578:dbl)
    n161 = Greater Or Equal?(x=w562, y=w573) -> (x >= y?=w577:bool)
    n162 = Bundle("Recording Time (min)"=w572, w578) -> (→"Trial Time Elapsed (Min)":cluster{"Recording Time (min)":dbl, dbl})  [unwired: 1 in]
    n163 = Write to Binary File(file (use dialog)=w547, data=w585, error in=w586, 5:FALSE ("prepend array or string size? (T)"), 9:T11."big-endian, network order" ("byte order (0:big-endian, network order)")) -> (refnum out=w582:refnum<file>, error out=w550:errorcluster)  [unwired: 1 in, 1 out]
    n164 = Replace Array Subset(array=w565, new element=w555, index=w557) -> (w564:bool[])
    "Solenoids" <- w564
    n165 = call-poly <vilib>:"DAQmx Write.vi"("task/channels in"=w569, "data"=w564, "error in"=w568) -> ("task out"=w567:refnum<k21>, "error out"=w566:errorcluster)  [unwired: 10 in, 1 out]
    n166 = local write "Stop"("Stop") -> ()
    n167 = Compound Arithmetic op=OR(w550, "Stop", w577) -> (w554:bool)
    "CBV Camera" <- w554
  }
  n168 = call <vilib>:"DAQmx Stop Task.vi"("task/channels in"=w240, "error in"=w1) -> ("task out"=w165:refnum<k21>, "error out"=w164:errorcluster)  [unwired: 12 in]
  n169 = call <vilib>:"IMAQ Extract Buffer.vi"("error in (no error)"=w318, "Buffer to extract"=-1, "IMAQ Session In"=w319) -> ("error out"=w340:errorcluster, "IMAQ Session Out"=w339:refnum<k11>)  [unwired: 7 out]
  n170 = Delete From Array(array=w226, length=1, index=0) -> (array with subset deleted=w21:u32[])  [unwired: 1 out]
  n171 = Close File(refnum=w317) -> (path=w220:path)  [unwired: 1 in, 1 out]
  n172 = Delete From Array(array=w70, length=1, index=0) -> (array with subset deleted=w20:u32[])  [unwired: 1 out]
  n173 = call-poly <vilib>:"DAQmx Write.vi"("task/channels in"=w54, "data"=FALSE, "error in"=w52) -> ("task out"=w51:refnum<k21>, "error out"=w49:errorcluster)  [unwired: 10 in, 1 out]
  n174 = call <vilib>:"DAQmx Stop Task.vi"("task/channels in"=w286, "error in"=w288) -> ()  [unwired: 12 in, 2 out]
  n175 = call <vilib>:"IMAQdx Close Camera.vi"("error in"=w163, "Session In"=w81) -> ()  [unwired: 9 in, 1 out]
  n176 = call "IMAQ AVI2 Close"("error in (no error)"=w290, "AVI Refnum"=w291) -> ("error out"=w219:errorcluster)  [unwired: 9 in]
  n177 = Close File(refnum=w285, error in=w163) -> (path=w218:path, error out=w217:errorcluster)
  n178 = call <vilib>:"IMAQdx Close Camera.vi"("error in"=w290, "Session In"=w292) -> ()  [unwired: 9 in, 1 out]
  n179 = call <vilib>:"DAQmx Clear Task.vi"("task in"=w165, "error in"=w164) -> ()  [unwired: 13 in, 1 out]
  n180 = Build Array(w20, w21) -> (w24:u32[][])
  n181 = call <vilib>:"DAQmx Stop Task.vi"("task/channels in"=w51, "error in"=w49) -> ("task out"=w50:refnum<k21>, "error out"=w48:errorcluster)  [unwired: 12 in]
  n182 = call <vilib>:"DAQmx Stop Task.vi"("task/channels in"=w188, "error in"=w187) -> ("task out"=w186:refnum<k21>, "error out"=w185:errorcluster)  [unwired: 12 in]
  n183 = call <vilib>:"DAQmx Stop Task.vi"("task/channels in"=w268, "error in"=w266) -> ()  [unwired: 12 in, 2 out]
  n184 = call <vilib>:"IMAQ Close.vi"("error in (no error)"=w340, "IMAQ Session In"=w339) -> ("error out"=w341:errorcluster)  [unwired: 9 out]
  n185 = Array To Spreadsheet String(delimiter (Tab)=",", array=w21, 3:"%d" ("format string")) -> (spreadsheet string=w74:string)
  n186 = Transpose 2D Array(2D array=w24) -> (transposed array=w23:u32[][])
  n187 = Array To Spreadsheet String(delimiter (Tab)=",", array=w20, 3:"%d" ("format string")) -> (spreadsheet string=w75:string)
  n188 = Move(source path=w3, error in=w219, 10:"Target Path") -> (error out=w214:errorcluster)  [unwired: 2 in, 2 out]
  n189 = call <vilib>:"DAQmx Clear Task.vi"("task in"=w50, "error in"=w48) -> ()  [unwired: 13 in, 1 out]
  n190 = for {
    N: w5 -> [_]
    tunnel: w335 -> [w609] mode=indexing
    shift-right: [w607] -> w222
    shift-left: w341 -> [w608]
    n191 = call "IMAQ Dispose"("All Images? (No)"=FALSE, "Image"=w609, "error in (no error)"=w608) -> ("error out"=w607:errorcluster)  [unwired: 3 out]
  }
  n192 = call <vilib>:"DAQmx Clear Task.vi"("task in"=w186, "error in"=w185) -> ()  [unwired: 13 in, 1 out]
  n193 = call <vilib>:"Trim Whitespace.vi"("string"=w75) -> ("trimmed string"=w72:string)  [unwired: 1 in]
  n194 = call <vilib>:"Trim Whitespace.vi"("string"=w74) -> ("trimmed string"=w73:string)  [unwired: 1 in]
  n195 = Number To Decimal String(number=w23) -> (decimal integer string=→"Dropped Frame Table":string[][])  [unwired: 1 in]
  n196 = Build Array(w72, w73) -> (w71:string[])
  n197 = call <vilib>:"Simple Error Handler.vi"("error in (no error)"=w214) -> ()  [unwired: 1 in, 8 out]
  n198 = Move(source path=w220, error in=w222, 10:"Target Path") -> (error out=w221:errorcluster)  [unwired: 2 in, 2 out]
  n199 = call <vilib>:"Simple Error Handler.vi"("error in (no error)"=w221) -> ()  [unwired: 1 in, 8 out]
  n200 = TDMS Set Properties(5:w71, 7:string[] ["WhiskerCam_DroppedFrameIndex", "WhiskerCam_NumberDropped"] ("channel name(s) in (Untitled)"), 8:w84, 11:w85) -> (0:w83:errorcluster, 3:w80:refnum<k34>)  [unwired: 2 in, 2 out]
  n201 = TDMS Close(8:w83, 11:w80) -> (0:w223:errorcluster, 3:w211:path)
  n202 = Path To String(path=w211) -> (string=w213:string)
  n203 = TDMS Defragment(4:w223, 7:w211) -> (0:w207:errorcluster)
  n204 = Concatenate Strings(w213, "_index" ("string")) -> (w210:string)
  n205 = Move(source path=w211, error in=w207, 10:"Target Path") -> (error out=w216:errorcluster)  [unwired: 2 in, 2 out]
  n206 = Move(source path=w218, error in=w217, 10:"Target Path") -> (error out=w215:errorcluster)  [unwired: 2 in, 2 out]
  n207 = String To Path(string=w210) -> (path=w209:path)
  n208 = call <vilib>:"Simple Error Handler.vi"("error in (no error)"=w215) -> ()  [unwired: 1 in, 8 out]
  n209 = call <vilib>:"Simple Error Handler.vi"("error in (no error)"=w216) -> ()  [unwired: 1 in, 8 out]
  n210 = Move(source path=w209, error in=w207, 10:"Target Path") -> ()  [unwired: 2 in, 3 out]
